vi "GenCM-Check Mandatory Connections.vi"(0 "Mandatory":T1, 5 "Analog":cluster{"Outputs":string[], "Inputs":string[]}[](array[cluster]), 9 "Digital":string[](array[string])) -> (15 "error out":errorcluster)   [LabVIEW 2015]
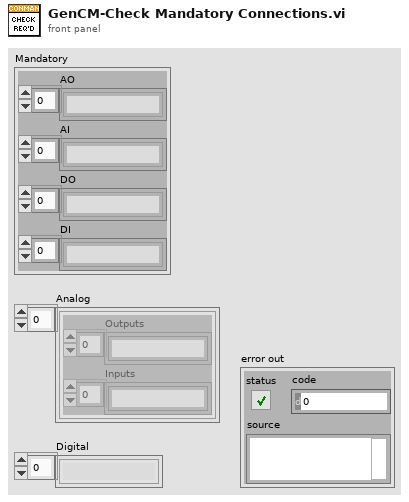
[diagram p1: front panel]
types:
  T1 = cluster{"AO":string[], "AI":string[], "DO":string[], "DI":string[]}
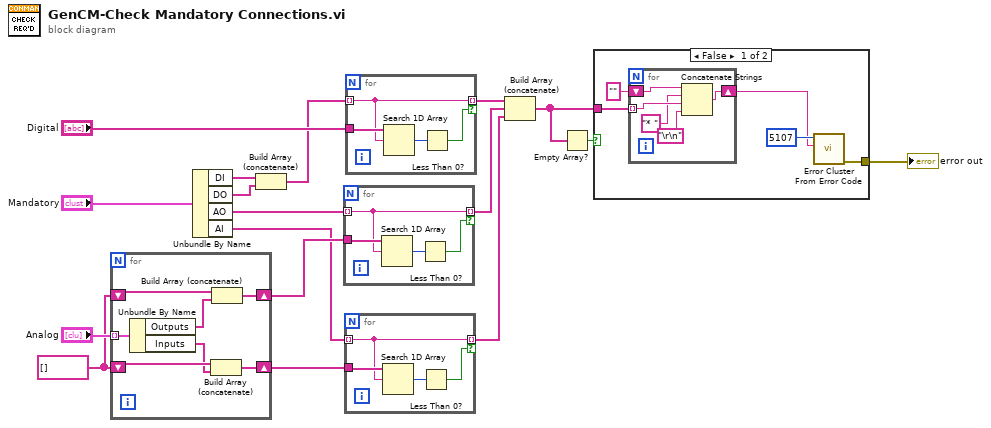
[diagram p0: block diagram]
diagram:
  w1 = string[] []
  n1 = for {
    tunnel: "Analog" -> [w24] mode=indexing
    shift-right: [w22] -> w14
    shift-left: w1 -> [w21]
    shift-right: [w20] -> w13
    shift-left: w1 -> [w19]
    n2 = Unbundle By Name(w24) -> ("Outputs"=w23:string[], "Inputs"=w18:string[])
    n3 = Build Array (concatenate)(w19, w18) -> (w20:string[])
    n4 = Build Array (concatenate)(w21, w23) -> (w22:string[])
  }
  n5 = Unbundle By Name("Mandatory") -> ("DI"=w10:string[], "DO"=w9:string[], "AO"=w15:string[], "AI"=w12:string[])
  n6 = Build Array (concatenate)(w10, w9) -> (w8:string[])
  n7 = for {
    tunnel: w15 -> [w27] mode=indexing
    tunnel: w14 -> [w28]
    tunnel: [w27] -> w6 mode=indexing if=w25
    n8 = Search 1D Array(1D array=w28, element=w27) -> (index of element=w26:i32)  [unwired: 1 in]
    n9 = Less Than 0?(x=w26) -> (x < 0?=w25:bool)
  }
  n10 = for {
    tunnel: w12 -> [w31] mode=indexing
    tunnel: w13 -> [w32]
    tunnel: [w31] -> w5 mode=indexing if=w29
    n11 = Search 1D Array(1D array=w32, element=w31) -> (index of element=w30:i32)  [unwired: 1 in]
    n12 = Less Than 0?(x=w30) -> (x < 0?=w29:bool)
  }
  n13 = for {
    tunnel: w8 -> [w35] mode=indexing
    tunnel: "Digital" -> [w36]
    tunnel: [w35] -> w7 mode=indexing if=w33
    n14 = Search 1D Array(1D array=w36, element=w35) -> (index of element=w34:i32)  [unwired: 1 in]
    n15 = Less Than 0?(x=w34) -> (x < 0?=w33:bool)
  }
  n16 = Build Array (concatenate)(w7, w6, w5) -> (w4:string[])
  n17 = Empty Array?(array=w4) -> (empty?=w3:bool)
  n18 = case shown="False" w3 {
    tunnel: w4 -> [w39 _]
    tunnel: [w40 _] -> w2
    frame False {
      n19 = for {
        tunnel: w39 -> [w44] mode=indexing
        shift-right: [w46] -> w37
        shift-left: "" -> [w45]
        n20 = Concatenate Strings(w45, "* ", w44, "\r\n") -> (w46:string)
      }
      n21 = call <vilib>:"Error Cluster From Error Code.vi"("error message (\"\")"=w37, "error code (0)"=5107 ("specific error code to clear (0: all)")) -> ("error out"=w40:errorcluster)  [unwired: 7 in]
    }
    frame True {
    }
  }
  "error out" <- w2
